vi "Write Customized File.vi"(8 "error in (no error)":errorcluster, 11 "Setup File in":refnum<class "Setup File.lvclass">) -> (0 "error out":errorcluster, 3 "Setup File out":refnum<class "Setup File.lvclass">)   [LabVIEW 2018, in "Setup File.lvclass"]
uses:
  Setup File.lvclass
  Setup File.lvclass/Setup File.ctl
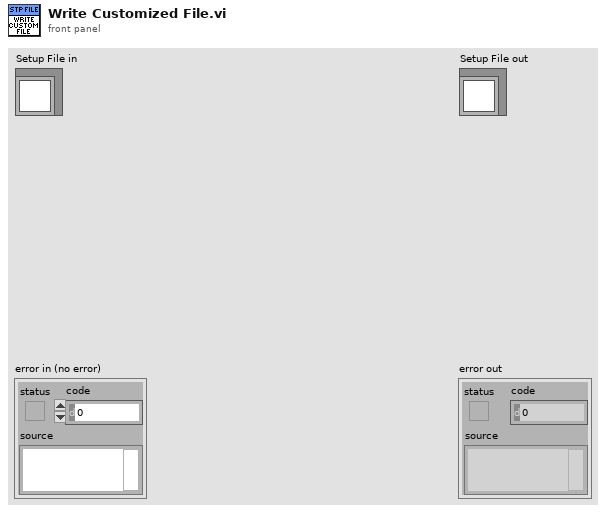
[diagram p1: front panel]
types:
  T1 = enum16{"open", "replace", "create", "open or create", "replace or create", "replace or create with confirmation"}
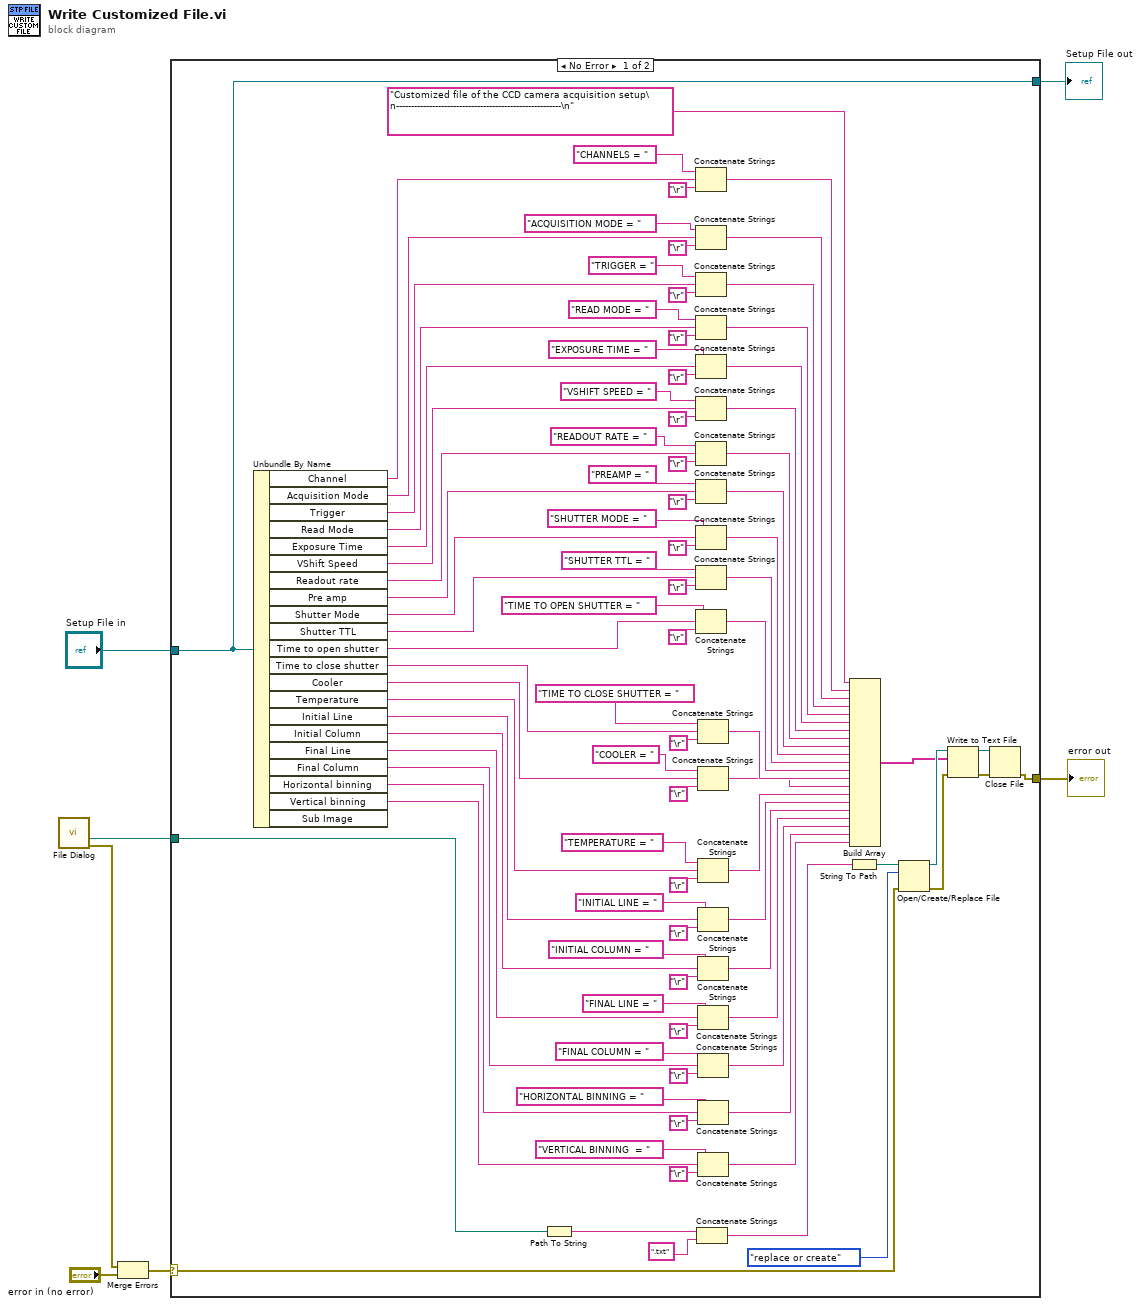
[diagram p0: block diagram]
diagram:
  n1 = call "File Dialog"() -> ("selected path"=w2:path, "error out"=w1:errorcluster)  [unwired: 12 in, 2 out]
  n2 = Merge Errors(w1, "error in (no error)") -> (w3:errorcluster)
  n3 = case shown="No Error" w3 {
    selector: w3 -> [w97 w104]
    tunnel: [w13 w104] -> w7
    tunnel: "Setup File in" -> [w59 w103]
    tunnel: [w59 w103] -> w6
    tunnel: w2 -> [w9 _]
    frame No Error {
      n4 = Unbundle By Name(w59) -> ("Channel"=w10:string, "Acquisition Mode"=w95:string, "Trigger"=w93:string, "Read Mode"=w91:string, "Exposure Time"=w89:string, "VShift Speed"=w87:string, "Readout rate"=w85:string, "Pre amp"=w83:string, "Shutter Mode"=w81:string, "Shutter TTL"=w80:string, "Time to open shutter"=w78:string, "Time to close shutter"=w76:string, "Cooler"=w74:string, "Temperature"=w72:string, "Initial Line"=w70:string, "Initial Column"=w68:string, "Final Line"=w66:string, "Final Column"=w64:string, "Horizontal binning"=w61:string, "Vertical binning"=w60:string)  [unwired: 1 out]
      n5 = Path To String(path=w9) -> (string=w37:string)
      n6 = Concatenate Strings("CHANNELS = ", w10, "\r") -> (w8:string)
      n7 = Concatenate Strings("ACQUISITION MODE = ", w95, "\r") -> (w57:string)
      n8 = Concatenate Strings("TRIGGER = ", w93, "\r") -> (w56:string)
      n9 = Concatenate Strings("READ MODE = ", w91, "\r") -> (w55:string)
      n10 = Concatenate Strings("EXPOSURE TIME = ", w89, "\r") -> (w54:string)
      n11 = Concatenate Strings("VSHIFT SPEED = ", w87, "\r") -> (w53:string)
      n12 = Concatenate Strings("READOUT RATE = ", w85, "\r") -> (w52:string)
      n13 = Concatenate Strings("PREAMP = ", w83, "\r") -> (w51:string)
      n14 = Concatenate Strings("SHUTTER MODE = ", w81, "\r") -> (w50:string)
      n15 = Concatenate Strings("SHUTTER TTL = ", w80, "\r") -> (w49:string)
      n16 = Concatenate Strings("TIME TO OPEN SHUTTER = ", w78, "\r") -> (w48:string)
      n17 = Concatenate Strings(w37, ".txt") -> (w35:string)
      n18 = Concatenate Strings("TIME TO CLOSE SHUTTER = ", w76, "\r") -> (w47:string)
      n19 = Concatenate Strings("COOLER = ", w74, "\r") -> (w46:string)
      n20 = Concatenate Strings("TEMPERATURE = ", w72, "\r") -> (w45:string)
      n21 = Concatenate Strings("INITIAL LINE = ", w70, "\r") -> (w44:string)
      n22 = Concatenate Strings("INITIAL COLUMN = ", w68, "\r") -> (w43:string)
      n23 = Concatenate Strings("FINAL LINE = ", w66, "\r") -> (w42:string)
      n24 = Concatenate Strings("FINAL COLUMN = ", w64, "\r") -> (w41:string)
      n25 = Concatenate Strings("HORIZONTAL BINNING = ", w61, "\r") -> (w40:string)
      n26 = Concatenate Strings("VERTICAL BINNING  = ", w60, "\r") -> (w39:string)
      n27 = String To Path(string=w35) -> (path=w34:path)
      n28 = Build Array("Customized file of the CCD camera acquisition setup\n-------------------------------------------------------\n" ("string"), w8, w57, w56, w55, w54, w53, w52, w51, w50, w49, w48, w47, w46, w45, w44, w43, w42, w41, w40, w39) -> (w38:string[])
      n29 = Open/Create/Replace File(file path (use dialog)=w34, error in=w97, operation (0:open)=T1."replace or create") -> (refnum out=w100:refnum<file>, error out=w102:errorcluster)  [unwired: 3 in, 1 out]
      n30 = Write to Text File(file (use dialog)=w100, text=w38, error in=w102) -> (refnum out=w99:refnum<file>, error out=w101:errorcluster)  [unwired: 1 in, 1 out]
      n31 = Close File(refnum=w99, error in=w101) -> (error out=w13:errorcluster)  [unwired: 1 out]
    }
    frame Error {
    }
  }
  "error out" <- w7
  "Setup File out" <- w6
